vi "OdometricNavigation.vi"(0 "Wheel Angles (rad)":T3 {"RR Angle (rad)" scale=3.1416..-3.1416; "RL Angle (rad)" scale=3.1416..-3.1416; "FR Angle (rad)" scale=3.1416..-3.1416; "FL Angle (rad)" scale=3.1416..-3.1416}, 1 "Wheel Movements (in.)":cluster{"FL":dbl, "FR":dbl, "RL":dbl, "RR":dbl} {"RR" scale=-70.0..70.0; "RL" scale=-70.0..70.0; "FR" scale=-70.0..70.0; "FL" scale=-70.0..70.0}, 2 "Robot angle (degrees)":dbl(knob) scale=180.0..-180.0, 3 "x and y error minimum (in.)":dbl, 4 "error minimum for rotation (rad)":dbl) -> (17 "movement":cluster{"sy":dbl, "sx":dbl, "rot.":dbl})   [LabVIEW 2014]
uses:
  <vilib>/Analysis/baseanly.llb/Mean (DBL).vi
  Robot Global Data.vi
  <vilib>/Analysis/NI_AALBase.lvlib
panel:
  out "unhandled error data":dbl[][](array[numeric])
  out "Wheel X movements":T1
  out "Wheel Y movements":T2
  out "1-side error rotation (rad)":dbl
  out "compared":cluster{"sy":dbl, "sx":dbl, "rot.":dbl}[](array[cluster])
  out "Right Error":bool
  out "Front Error":bool
  out "Rear Error":bool
  out "Left Error":bool
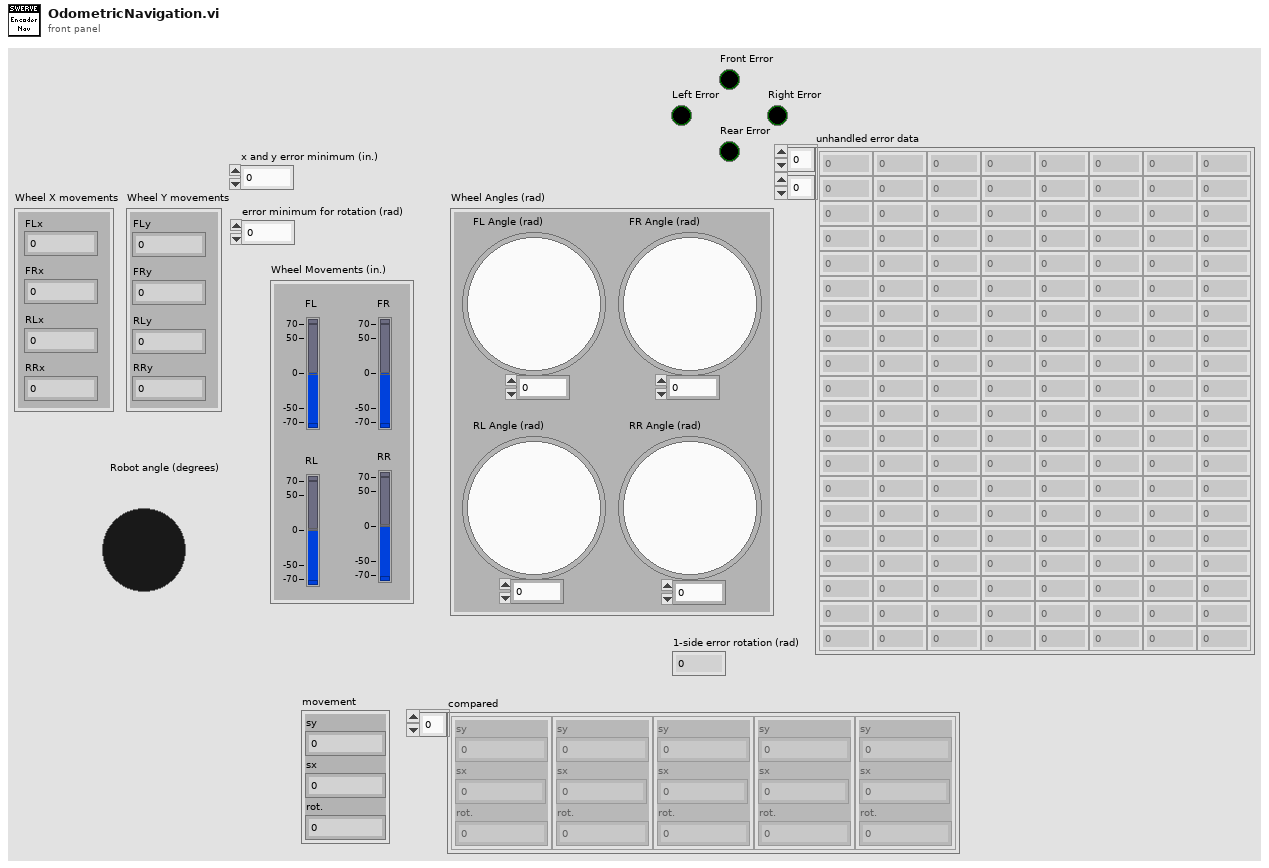
[diagram p1: front panel]
types:
  T1 = cluster{"FLx":dbl, "FRx":dbl, "RLx":dbl, "RRx":dbl}
  T2 = cluster{"FLy":dbl, "FRy":dbl, "RLy":dbl, "RRy":dbl}
  T3 = cluster{"FL Angle (rad)":dbl, "FR Angle (rad)":dbl, "RL Angle (rad)":dbl, "RR Angle (rad)":dbl}
  T4 = cluster{"[0]":dbl, "[1]":dbl, "[2]":dbl, "[3]":dbl}
  T5 = enum16{"no error", "front", "rear", "left", "right", "FL", "FR", "RL", "RR", "other"}
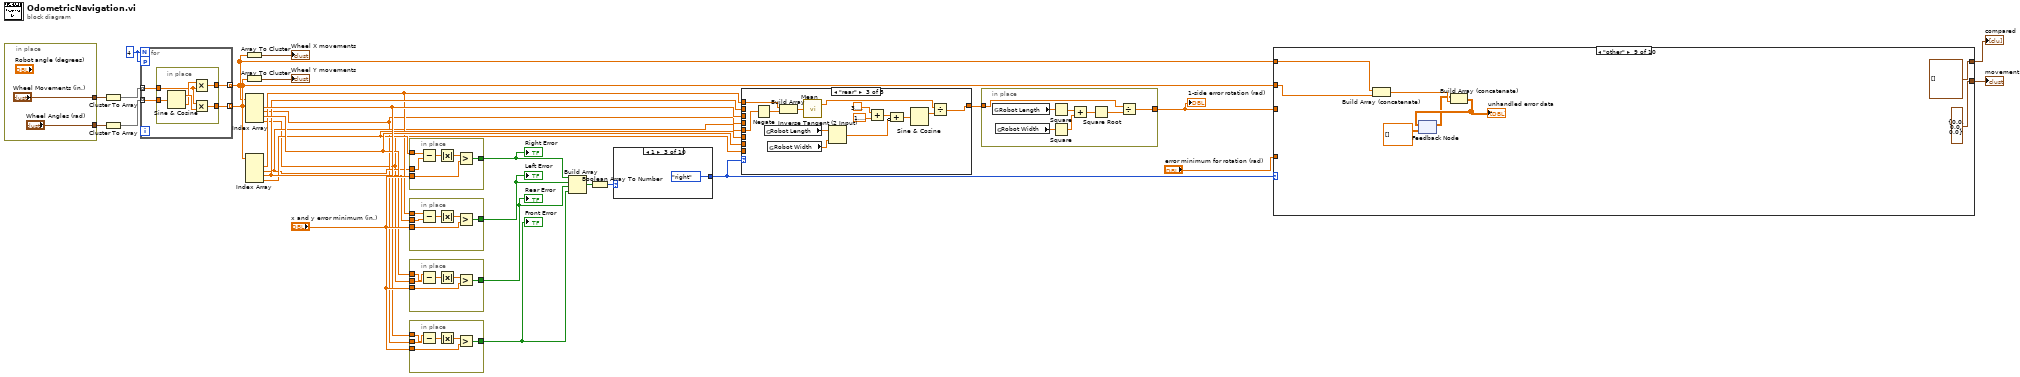
[diagram p0: block diagram]
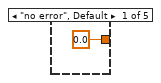
[diagram p2: hidden frame]
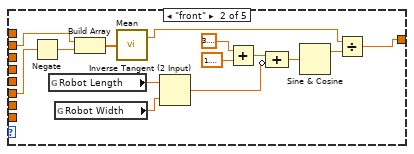
[diagram p3: hidden frame]
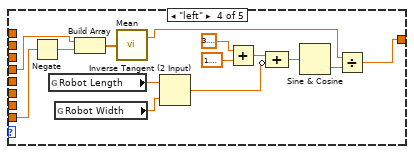
[diagram p4: hidden frame]
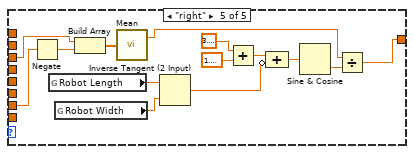
[diagram p5: hidden frame]
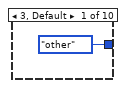
[diagram p6: hidden frame]
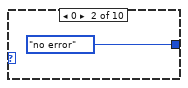
[diagram p7: hidden frame]
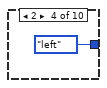
[diagram p8: hidden frame]
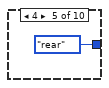
[diagram p9: hidden frame]
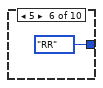
[diagram p10: hidden frame]
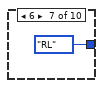
[diagram p11: hidden frame]
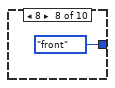
[diagram p12: hidden frame]
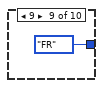
[diagram p13: hidden frame]
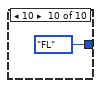
[diagram p14: hidden frame]
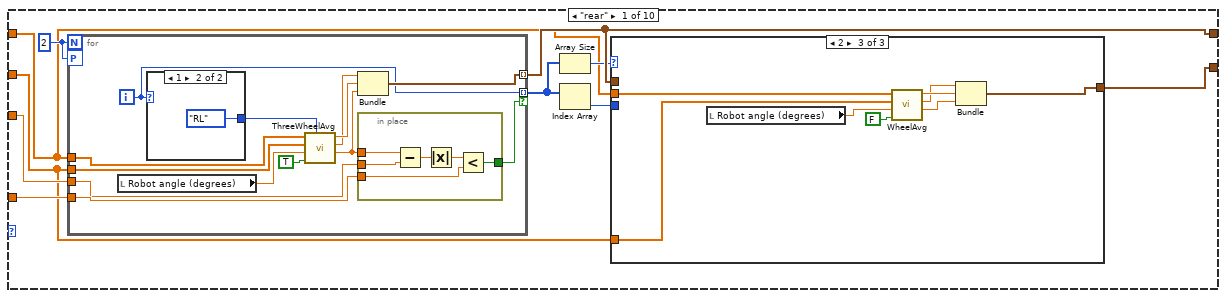
[diagram p15: hidden frame]
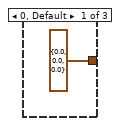
[diagram p16: hidden frame]
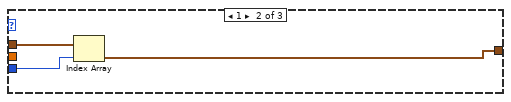
[diagram p17: hidden frame]
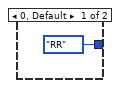
[diagram p18: hidden frame]
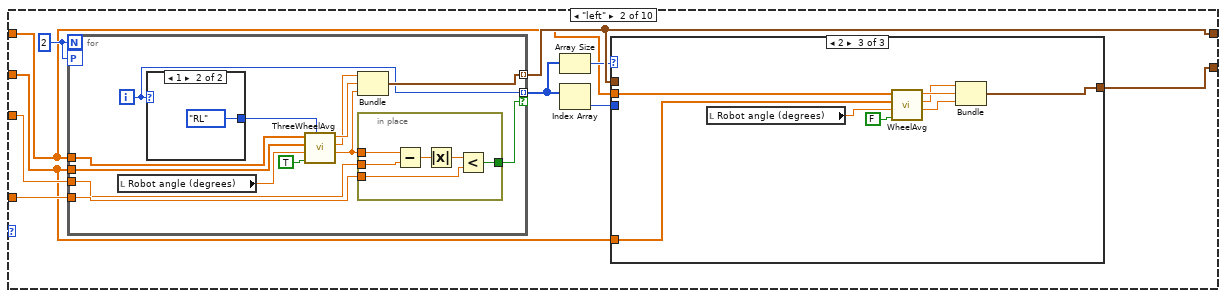
[diagram p19: hidden frame]
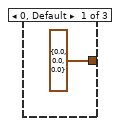
[diagram p20: hidden frame]
diagram:
  w16 = 4
  n1 = in-place {
    in-place-border: ["Wheel Movements (in.)"] -> w19
    in-place-border: ["Wheel Angles (rad)"] -> w18
  }
  n2 = Cluster To Array(cluster=w19) -> (array=w20:dbl[])
  n3 = Cluster To Array(cluster=w18) -> (array=w17:dbl[])
  n4 = for {
    N: w16 -> [_]
    tunnel: w20 -> [w36] mode=indexing
    tunnel: w17 -> [w35] mode=indexing
    workers-P: w16 -> [_]
    tunnel: [w34] -> w3 mode=indexing
    tunnel: [w33] -> w2 mode=indexing
    n5 = in-place {
      in-place-border: [w40] -> w33
      in-place-border: [w39] -> w34
      in-place-border: w36 -> [w38]
      in-place-border: w35 -> [w37]
      n6 = Sine & Cosine(0:w37) -> (1:w42:dbl, 2:w41:dbl)
      n7 = Multiply(x=w41, y=w38) -> (x*y=w40:dbl)
      n8 = Multiply(x=w38, y=w42) -> (x*y=w39:dbl)
    }
  }
  n9 = Array To Cluster(array=w2) -> (cluster=→"Wheel X movements":T4)
  n10 = Array To Cluster(array=w3) -> (cluster=→"Wheel Y movements":T4)
  n11 = Index Array(array=w2) -> (element #1=w12:dbl, element #2=w6:dbl, element #3=w11:dbl, element #4=w5:dbl)  [unwired: 4 in]
  n12 = Index Array(array=w3) -> (element #1=w8:dbl, element #2=w7:dbl, element #3=w10:dbl, element #4=w9:dbl)  [unwired: 4 in]
  n13 = in-place {
    in-place-border: [w46] -> w24
    in-place-border: w9 -> [w45]
    in-place-border: w7 -> [w44]
    in-place-border: "x and y error minimum (in.)" -> [w43]
    n14 = Subtract(x=w45, y=w44) -> (x-y=w48:dbl)
    n15 = Absolute Value(x=w48) -> (abs(x)=w47:dbl)
    n16 = Greater?(x=w47, y=w43) -> (0:w46:bool)
  }
  "Right Error" <- w24
  n17 = in-place {
    in-place-border: [w52] -> w21
    in-place-border: w8 -> [w51]
    in-place-border: w10 -> [w50]
    in-place-border: "x and y error minimum (in.)" -> [w49]
    n18 = Subtract(x=w51, y=w50) -> (x-y=w54:dbl)
    n19 = Absolute Value(x=w54) -> (abs(x)=w53:dbl)
    n20 = Greater?(x=w53, y=w49) -> (0:w52:bool)
  }
  "Left Error" <- w21
  n21 = in-place {
    in-place-border: [w58] -> w22
    in-place-border: w5 -> [w57]
    in-place-border: w11 -> [w56]
    in-place-border: "x and y error minimum (in.)" -> [w55]
    n22 = Subtract(x=w57, y=w56) -> (x-y=w60:dbl)
    n23 = Absolute Value(x=w60) -> (abs(x)=w59:dbl)
    n24 = Greater?(x=w59, y=w55) -> (0:w58:bool)
  }
  "Rear Error" <- w22
  n25 = in-place {
    in-place-border: [w64] -> w23
    in-place-border: w6 -> [w63]
    in-place-border: w12 -> [w62]
    in-place-border: "x and y error minimum (in.)" -> [w61]
    n26 = Subtract(x=w63, y=w62) -> (x-y=w66:dbl)
    n27 = Absolute Value(x=w66) -> (abs(x)=w65:dbl)
    n28 = Greater?(x=w65, y=w61) -> (0:w64:bool)
  }
  "Front Error" <- w23
  n29 = Build Array(w24, w21, w22, w23) -> (w26:bool[])
  n30 = Boolean Array To Number(Boolean array=w26) -> (number=w25:u32)
  n31 = case shown="1" w25 {
    tunnel: [T5."other" T5."no error" T5."right" T5."left" T5."rear" T5."RR" T5."RL" T5."front" T5."FR" T5."FL"] -> w13
    frame 3, Default {
    }
    frame 0 {
    }
    frame 1 {
    }
    frame 2 {
    }
    frame 4 {
    }
    frame 5 {
    }
    frame 6 {
    }
    frame 8 {
    }
    frame 9 {
    }
    frame 10 {
    }
  }
  n32 = case shown="\"rear\"" w13 {
    tunnel: [0.0 w80 w92 w106 w122] -> w4
    tunnel: w12 -> [_ _ _ _ w121]
    tunnel: w11 -> [_ _ _ _ w120]
    tunnel: w10 -> [_ w79 _ _ _]
    tunnel: w9 -> [_ w78 _ _ _]
    tunnel: w8 -> [_ _ w95 _ _]
    tunnel: w7 -> [_ _ w94 _ _]
    tunnel: w6 -> [_ _ _ w108 _]
    tunnel: w5 -> [_ _ _ w107 _]
    frame "no error", Default {
    }
    frame "front" {
      n33 = Negate(x=w78) -> (-x=w90:dbl)
      n34 = global read "Robot Global Data.vi" "Robot Length"() -> (w83:dbl)
      n35 = global read "Robot Global Data.vi" "Robot Width"() -> (w84:dbl)
      n36 = Build Array(w79, w90) -> (w91:dbl[])
      n37 = call-poly <vilib>:"Mean.vi"("X"=w91) -> ("mean"=w89:dbl)  [unwired: 1 out]
      n38 = Inverse Tangent (2 Input)(1:w84, 2:w83) -> (0:w85:dbl)
      n39 = Add(x=3.141592653589793, y=1.5707963267948966) -> (x+y=w86:dbl)
      n40 = Compound Arithmetic op=ADD(w86, invert w85) -> (w82:dbl)
      n41 = Sine & Cosine(0:w82) -> (1:w81:dbl)  [unwired: 1 out]
      n42 = Divide(x=w89, y=w81) -> (x/y=w80:dbl)
    }
    frame "rear" {
      n43 = Negate(x=w94) -> (-x=w104:dbl)
      n44 = global read "Robot Global Data.vi" "Robot Length"() -> (w98:dbl)
      n45 = global read "Robot Global Data.vi" "Robot Width"() -> (w99:dbl)
      n46 = Build Array(w95, w104) -> (w105:dbl[])
      n47 = call-poly <vilib>:"Mean.vi"("X"=w105) -> ("mean"=w103:dbl)  [unwired: 1 out]
      n48 = Inverse Tangent (2 Input)(1:w99, 2:w98) -> (0:w93:dbl)
      n49 = Add(x=3.141592653589793, y=1.5707963267948966) -> (x+y=w100:dbl)
      n50 = Compound Arithmetic op=ADD(w100, invert w93) -> (w97:dbl)
      n51 = Sine & Cosine(0:w97) -> (1:w96:dbl)  [unwired: 1 out]
      n52 = Divide(x=w103, y=w96) -> (x/y=w92:dbl)
    }
    frame "left" {
      n53 = Negate(x=w107) -> (-x=w118:dbl)
      n54 = global read "Robot Global Data.vi" "Robot Length"() -> (w111:dbl)
      n55 = global read "Robot Global Data.vi" "Robot Width"() -> (w112:dbl)
      n56 = Build Array(w108, w118) -> (w119:dbl[])
      n57 = call-poly <vilib>:"Mean.vi"("X"=w119) -> ("mean"=w117:dbl)  [unwired: 1 out]
      n58 = Inverse Tangent (2 Input)(1:w112, 2:w111) -> (0:w113:dbl)
      n59 = Add(x=3.141592653589793, y=1.5707963267948966) -> (x+y=w114:dbl)
      n60 = Compound Arithmetic op=ADD(w114, invert w113) -> (w110:dbl)
      n61 = Sine & Cosine(0:w110) -> (2:w109:dbl)  [unwired: 1 out]
      n62 = Divide(x=w117, y=w109) -> (x/y=w106:dbl)
    }
    frame "right" {
      n63 = Negate(x=w120) -> (-x=w132:dbl)
      n64 = global read "Robot Global Data.vi" "Robot Length"() -> (w126:dbl)
      n65 = global read "Robot Global Data.vi" "Robot Width"() -> (w127:dbl)
      n66 = Build Array(w121, w132) -> (w133:dbl[])
      n67 = call-poly <vilib>:"Mean.vi"("X"=w133) -> ("mean"=w124:dbl)  [unwired: 1 out]
      n68 = Inverse Tangent (2 Input)(1:w127, 2:w126) -> (0:w128:dbl)
      n69 = Add(x=3.141592653589793, y=1.5707963267948966) -> (x+y=w129:dbl)
      n70 = Compound Arithmetic op=ADD(w129, invert w128) -> (w125:dbl)
      n71 = Sine & Cosine(0:w125) -> (2:w123:dbl)  [unwired: 1 out]
      n72 = Divide(x=w124, y=w123) -> (x/y=w122:dbl)
    }
  }
  n73 = in-place {
    in-place-border: w4 -> [w135]
    in-place-border: [w134] -> w1
    n74 = global read "Robot Global Data.vi" "Robot Length"() -> (w141:dbl)
    n75 = global read "Robot Global Data.vi" "Robot Width"() -> (w140:dbl)
    n76 = Square(x=w141) -> (x^2=w138:dbl)
    n77 = Square(x=w140) -> (x^2=w139:dbl)
    n78 = Add(x=w138, y=w139) -> (x+y=w137:dbl)
    n79 = Square Root(x=w137) -> (sqrt(x)=w136:dbl)
    n80 = Divide(x=w135, y=w136) -> (x/y=w134:dbl)
  }
  "1-side error rotation (rad)" <- w1
  n81 = case shown="\"other\"" w13 {
    tunnel: [w147 w190 w233 w276 cluster{"mean":dbl, "mean":dbl, "mean":dbl}[] [] cluster{"mean":dbl, "mean":dbl, "mean":dbl}[] [] cluster{"mean":dbl, "mean":dbl, "mean":dbl}[] [] cluster{"mean":dbl, "mean":dbl, "mean":dbl}[] [] cluster{"mean":dbl, "mean":dbl, "mean":dbl}[] [] cluster{"mean":dbl, "mean":dbl, "mean":dbl}[] []] -> w29
    tunnel: "error minimum for rotation (rad)" -> [w151 w194 w237 w280 _ _ _ _ _ _]
    tunnel: [w148 w191 w234 w277 w323 w333 w343 w353 cluster{"mean":dbl, "mean":dbl, "mean":dbl} {"mean"=0.0, "mean"=0.0, "mean"=0.0} w369] -> w27
    tunnel: w3 -> [w143 w186 w229 w272 w319 w329 w339 w349 w358 w364]
    tunnel: w2 -> [w142 w185 w228 w271 w318 w328 w338 w348 w359 w363]
    tunnel: w1 -> [w146 w189 w232 w275 _ _ _ _ _ _]
    frame "rear" {
      w145 = 2
      n82 = for {
        N: w145 -> [_]
        tunnel: [w176] -> w147 mode=indexing
        tunnel: w151 -> [w175]
        tunnel: [w174] -> w150 mode=indexing if=w173
        tunnel: w143 -> [w170]
        tunnel: w142 -> [w169]
        tunnel: w146 -> [w164]
        workers-P: w145 -> [_]
        i -> [w174]
        n83 = local read "Robot angle (degrees)"() -> (w171:dbl)
        n84 = case shown="1" w174 {
          tunnel: [enum16{"FL", "FR", "RL", "RR"}."RR" ("Wheel Missing") enum16{"FL", "FR", "RL", "RR"}."RL" ("Wheel Missing")] -> w168
          frame 0, Default {
          }
          frame 1 {
          }
        }
        n85 = call "ThreeWheelAvg.vi"("Wheel Missing"=w168, "Calculate Rotation?"=TRUE, "Robot Angle (degrees)"=w171, "wheel Y movements (FL, FR, RL, RR)"=w170, "wheel X movements (FL, FR, RL, RR)"=w169) -> ("Rotation"=w165:dbl, "Y"=w166:dbl, "X"=w167:dbl)  [unwired: 4 in]
        n86 = Bundle("Y"=w166, "X"=w167, "Rotation"=w165) -> (w176:cluster{"Y":dbl, "X":dbl, "Rotation":dbl})  [unwired: 1 in]
        n87 = in-place {
          in-place-border: [w180] -> w173
          in-place-border: w175 -> [w179]
          in-place-border: w165 -> [w178]
          in-place-border: w164 -> [w177]
          n88 = Subtract(x=w178, y=w177) -> (x-y=w182:dbl)
          n89 = Absolute Value(x=w182) -> (abs(x)=w181:dbl)
          n90 = Less?(x=w181, y=w179) -> (x < y?=w180:bool)
        }
      }
      n91 = Array Size(array=w150) -> (size(s)=w144:i32)
      n92 = Index Array(array=w150) -> (element=w149:i32)  [unwired: 1 in]
      n93 = case shown="2" w144 {
        tunnel: w149 -> [_ w153 _]
        tunnel: [cluster{"Y":dbl, "X":dbl, "Rotation":dbl} {"Y"=0.0, "X"=0.0, "Rotation"=0.0} w155 w158] -> w148
        tunnel: w147 -> [_ w154 _]
        tunnel: w143 -> [_ _ w163]
        tunnel: w142 -> [_ _ w162]
        frame 0, Default {
        }
        frame 1 {
          n94 = Index Array(array=w154, index=w153) -> (element=w155:cluster{"Y":dbl, "X":dbl, "Rotation":dbl})
        }
        frame 2 {
          n95 = local read "Robot angle (degrees)"() -> (w156:dbl)
          n96 = call "WheelAvg.vi"("Calculate Rotation?"=FALSE, "Robot Angle (degrees)"=w156, "wheel Y movements (FL, FR, RL, RR)"=w163, "wheel X movements (FL, FR, RL, RR)"=w162) -> ("Rotation"=w159:dbl, "Y"=w160:dbl, "X"=w161:dbl)  [unwired: 5 in]
          n97 = Bundle("Y"=w160, "X"=w161, "Rotation"=w159) -> (w158:cluster{"Y":dbl, "X":dbl, "Rotation":dbl})  [unwired: 1 in]
        }
      }
    }
    frame "left" {
      w188 = 2
      n98 = for {
        N: w188 -> [_]
        tunnel: [w219] -> w190 mode=indexing
        tunnel: w194 -> [w218]
        tunnel: [w217] -> w193 mode=indexing if=w216
        tunnel: w186 -> [w213]
        tunnel: w185 -> [w212]
        tunnel: w189 -> [w207]
        workers-P: w188 -> [_]
        i -> [w217]
        n99 = local read "Robot angle (degrees)"() -> (w214:dbl)
        n100 = case shown="1" w217 {
          tunnel: [enum16{"FL", "FR", "RL", "RR"}."RR" ("Wheel Missing") enum16{"FL", "FR", "RL", "RR"}."RL" ("Wheel Missing")] -> w211
          frame 0, Default {
          }
          frame 1 {
          }
        }
        n101 = call "ThreeWheelAvg.vi"("Wheel Missing"=w211, "Calculate Rotation?"=TRUE, "Robot Angle (degrees)"=w214, "wheel Y movements (FL, FR, RL, RR)"=w213, "wheel X movements (FL, FR, RL, RR)"=w212) -> ("Rotation"=w208:dbl, "Y"=w209:dbl, "X"=w210:dbl)  [unwired: 4 in]
        n102 = Bundle("Y"=w209, "X"=w210, "Rotation"=w208) -> (w219:cluster{"Y":dbl, "X":dbl, "Rotation":dbl})  [unwired: 1 in]
        n103 = in-place {
          in-place-border: [w223] -> w216
          in-place-border: w218 -> [w222]
          in-place-border: w208 -> [w221]
          in-place-border: w207 -> [w220]
          n104 = Subtract(x=w221, y=w220) -> (x-y=w225:dbl)
          n105 = Absolute Value(x=w225) -> (abs(x)=w224:dbl)
          n106 = Less?(x=w224, y=w222) -> (x < y?=w223:bool)
        }
      }
      n107 = Array Size(array=w193) -> (size(s)=w187:i32)
      n108 = Index Array(array=w193) -> (element=w192:i32)  [unwired: 1 in]
      n109 = case shown="2" w187 {
        tunnel: w192 -> [_ w196 _]
        tunnel: [cluster{"Y":dbl, "X":dbl, "Rotation":dbl} {"Y"=0.0, "X"=0.0, "Rotation"=0.0} w198 w201] -> w191
        tunnel: w190 -> [_ w197 _]
        tunnel: w186 -> [_ _ w206]
        tunnel: w185 -> [_ _ w205]
        frame 0, Default {
        }
        frame 1 {
          n110 = Index Array(array=w197, index=w196) -> (element=w198:cluster{"Y":dbl, "X":dbl, "Rotation":dbl})
        }
        frame 2 {
          n111 = local read "Robot angle (degrees)"() -> (w199:dbl)
          n112 = call "WheelAvg.vi"("Calculate Rotation?"=FALSE, "Robot Angle (degrees)"=w199, "wheel Y movements (FL, FR, RL, RR)"=w206, "wheel X movements (FL, FR, RL, RR)"=w205) -> ("Rotation"=w202:dbl, "Y"=w203:dbl, "X"=w204:dbl)  [unwired: 5 in]
          n113 = Bundle("Y"=w203, "X"=w204, "Rotation"=w202) -> (w201:cluster{"Y":dbl, "X":dbl, "Rotation":dbl})  [unwired: 1 in]
        }
      }
    }
    frame "right" {
      w231 = 2
      n114 = for {
        N: w231 -> [_]
        tunnel: [w262] -> w233 mode=indexing
        tunnel: w237 -> [w261]
        tunnel: [w260] -> w236 mode=indexing if=w259
        tunnel: w229 -> [w256]
        tunnel: w228 -> [w255]
        tunnel: w232 -> [w250]
        workers-P: w231 -> [_]
        i -> [w260]
        n115 = local read "Robot angle (degrees)"() -> (w257:dbl)
        n116 = case shown="1" w260 {
          tunnel: [enum16{"FL", "FR", "RL", "RR"}."RR" ("Wheel Missing") enum16{"FL", "FR", "RL", "RR"}."RL" ("Wheel Missing")] -> w254
          frame 0, Default {
          }
          frame 1 {
          }
        }
        n117 = call "ThreeWheelAvg.vi"("Wheel Missing"=w254, "Calculate Rotation?"=TRUE, "Robot Angle (degrees)"=w257, "wheel Y movements (FL, FR, RL, RR)"=w256, "wheel X movements (FL, FR, RL, RR)"=w255) -> ("Rotation"=w251:dbl, "Y"=w252:dbl, "X"=w253:dbl)  [unwired: 4 in]
        n118 = Bundle("Y"=w252, "X"=w253, "Rotation"=w251) -> (w262:cluster{"Y":dbl, "X":dbl, "Rotation":dbl})  [unwired: 1 in]
        n119 = in-place {
          in-place-border: [w266] -> w259
          in-place-border: w261 -> [w265]
          in-place-border: w251 -> [w264]
          in-place-border: w250 -> [w263]
          n120 = Subtract(x=w264, y=w263) -> (x-y=w268:dbl)
          n121 = Absolute Value(x=w268) -> (abs(x)=w267:dbl)
          n122 = Less?(x=w267, y=w265) -> (x < y?=w266:bool)
        }
      }
      n123 = Array Size(array=w236) -> (size(s)=w230:i32)
      n124 = Index Array(array=w236) -> (element=w235:i32)  [unwired: 1 in]
      n125 = case shown="2" w230 {
        tunnel: w235 -> [_ w239 _]
        tunnel: [cluster{"Y":dbl, "X":dbl, "Rotation":dbl} {"Y"=0.0, "X"=0.0, "Rotation"=0.0} w241 w244] -> w234
        tunnel: w233 -> [_ w240 _]
        tunnel: w229 -> [_ _ w249]
        tunnel: w228 -> [_ _ w248]
        frame 0, Default {
        }
        frame 1 {
          n126 = Index Array(array=w240, index=w239) -> (element=w241:cluster{"Y":dbl, "X":dbl, "Rotation":dbl})
        }
        frame 2 {
          n127 = local read "Robot angle (degrees)"() -> (w242:dbl)
          n128 = call "WheelAvg.vi"("Calculate Rotation?"=FALSE, "Robot Angle (degrees)"=w242, "wheel Y movements (FL, FR, RL, RR)"=w249, "wheel X movements (FL, FR, RL, RR)"=w248) -> ("Rotation"=w245:dbl, "Y"=w246:dbl, "X"=w247:dbl)  [unwired: 5 in]
          n129 = Bundle("Y"=w246, "X"=w247, "Rotation"=w245) -> (w244:cluster{"Y":dbl, "X":dbl, "Rotation":dbl})  [unwired: 1 in]
        }
      }
    }
    frame "front" {
      w274 = 2
      n130 = for {
        N: w274 -> [_]
        tunnel: [w305] -> w276 mode=indexing
        tunnel: w280 -> [w304]
        tunnel: [w303] -> w279 mode=indexing if=w302
        tunnel: w272 -> [w299]
        tunnel: w271 -> [w298]
        tunnel: w275 -> [w293]
        workers-P: w274 -> [_]
        i -> [w303]
        n131 = local read "Robot angle (degrees)"() -> (w300:dbl)
        n132 = case shown="1" w303 {
          tunnel: [enum16{"FL", "FR", "RL", "RR"}."RR" ("Wheel Missing") enum16{"FL", "FR", "RL", "RR"}."RL" ("Wheel Missing")] -> w297
          frame 0, Default {
          }
          frame 1 {
          }
        }
        n133 = call "ThreeWheelAvg.vi"("Wheel Missing"=w297, "Calculate Rotation?"=TRUE, "Robot Angle (degrees)"=w300, "wheel Y movements (FL, FR, RL, RR)"=w299, "wheel X movements (FL, FR, RL, RR)"=w298) -> ("Rotation"=w294:dbl, "Y"=w295:dbl, "X"=w296:dbl)  [unwired: 4 in]
        n134 = Bundle("Y"=w295, "X"=w296, "Rotation"=w294) -> (w305:cluster{"Y":dbl, "X":dbl, "Rotation":dbl})  [unwired: 1 in]
        n135 = in-place {
          in-place-border: [w309] -> w302
          in-place-border: w304 -> [w308]
          in-place-border: w294 -> [w307]
          in-place-border: w293 -> [w306]
          n136 = Subtract(x=w307, y=w306) -> (x-y=w311:dbl)
          n137 = Absolute Value(x=w311) -> (abs(x)=w310:dbl)
          n138 = Less?(x=w310, y=w308) -> (x < y?=w309:bool)
        }
      }
      n139 = Array Size(array=w279) -> (size(s)=w273:i32)
      n140 = Index Array(array=w279) -> (element=w278:i32)  [unwired: 1 in]
      n141 = case shown="2" w273 {
        tunnel: w278 -> [_ w282 _]
        tunnel: [cluster{"Y":dbl, "X":dbl, "Rotation":dbl} {"Y"=0.0, "X"=0.0, "Rotation"=0.0} w284 w287] -> w277
        tunnel: w276 -> [_ w283 _]
        tunnel: w272 -> [_ _ w292]
        tunnel: w271 -> [_ _ w291]
        frame 0, Default {
        }
        frame 1 {
          n142 = Index Array(array=w283, index=w282) -> (element=w284:cluster{"Y":dbl, "X":dbl, "Rotation":dbl})
        }
        frame 2 {
          n143 = local read "Robot angle (degrees)"() -> (w285:dbl)
          n144 = call "WheelAvg.vi"("Calculate Rotation?"=FALSE, "Robot Angle (degrees)"=w285, "wheel Y movements (FL, FR, RL, RR)"=w292, "wheel X movements (FL, FR, RL, RR)"=w291) -> ("Rotation"=w288:dbl, "Y"=w289:dbl, "X"=w290:dbl)  [unwired: 5 in]
          n145 = Bundle("Y"=w289, "X"=w290, "Rotation"=w288) -> (w287:cluster{"Y":dbl, "X":dbl, "Rotation":dbl})  [unwired: 1 in]
        }
      }
    }
    frame "FL" {
      # "fl"
      n146 = local read "Robot angle (degrees)"() -> (w321:dbl)
      n147 = call "ThreeWheelAvg.vi"("Wheel Missing"=enum16{"FL", "FR", "RL", "RR"}."FL", "Calculate Rotation?"=FALSE, "Robot Angle (degrees)"=w321, "wheel Y movements (FL, FR, RL, RR)"=w319, "wheel X movements (FL, FR, RL, RR)"=w318) -> ("Rotation"=w315:dbl, "Y"=w314:dbl, "X"=w316:dbl)  [unwired: 4 in]
      n148 = Bundle("Y"=w314, "X"=w316, "Rotation"=w315) -> (w323:cluster{"Y":dbl, "X":dbl, "Rotation":dbl})  [unwired: 1 in]
    }
    frame "FR" {
      # "fl"
      n149 = local read "Robot angle (degrees)"() -> (w331:dbl)
      n150 = call "ThreeWheelAvg.vi"("Wheel Missing"=enum16{"FL", "FR", "RL", "RR"}."FR", "Calculate Rotation?"=FALSE, "Robot Angle (degrees)"=w331, "wheel Y movements (FL, FR, RL, RR)"=w329, "wheel X movements (FL, FR, RL, RR)"=w328) -> ("Rotation"=w325:dbl, "Y"=w324:dbl, "X"=w326:dbl)  [unwired: 4 in]
      n151 = Bundle("Y"=w324, "X"=w326, "Rotation"=w325) -> (w333:cluster{"Y":dbl, "X":dbl, "Rotation":dbl})  [unwired: 1 in]
    }
    frame "RL" {
      # "fl"
      n152 = local read "Robot angle (degrees)"() -> (w341:dbl)
      n153 = call "ThreeWheelAvg.vi"("Wheel Missing"=enum16{"FL", "FR", "RL", "RR"}."RL", "Calculate Rotation?"=FALSE, "Robot Angle (degrees)"=w341, "wheel Y movements (FL, FR, RL, RR)"=w339, "wheel X movements (FL, FR, RL, RR)"=w338) -> ("Rotation"=w335:dbl, "Y"=w334:dbl, "X"=w336:dbl)  [unwired: 4 in]
      n154 = Bundle("Y"=w334, "X"=w336, "Rotation"=w335) -> (w343:cluster{"Y":dbl, "X":dbl, "Rotation":dbl})  [unwired: 1 in]
    }
    frame "RR" {
      # "fl"
      n155 = local read "Robot angle (degrees)"() -> (w351:dbl)
      n156 = call "ThreeWheelAvg.vi"("Wheel Missing"=enum16{"FL", "FR", "RL", "RR"}."RR", "Calculate Rotation?"=FALSE, "Robot Angle (degrees)"=w351, "wheel Y movements (FL, FR, RL, RR)"=w349, "wheel X movements (FL, FR, RL, RR)"=w348) -> ("Rotation"=w345:dbl, "Y"=w344:dbl, "X"=w346:dbl)  [unwired: 4 in]
      n157 = Bundle("Y"=w344, "X"=w346, "Rotation"=w345) -> (w353:cluster{"Y":dbl, "X":dbl, "Rotation":dbl})  [unwired: 1 in]
    }
    frame "other" {
      n158 = Build Array (concatenate)(w359, w358) -> (w357:dbl[])
      n159 = feedback #1(dbl[][] []) -> (w355:dbl[][])
      n160 = Build Array (concatenate)(w355, w357) -> (w356:dbl[][])
      "unhandled error data" <- w356
      n161 = feedback-in #1(w356) -> ()
    }
    frame "no error" {
      n162 = local read "Robot angle (degrees)"() -> (w362:dbl)
      n163 = call "WheelAvg.vi"("Calculate Rotation?"=FALSE, "Robot Angle (degrees)"=w362, "wheel Y movements (FL, FR, RL, RR)"=w364, "wheel X movements (FL, FR, RL, RR)"=w363) -> ("Rotation"=w366:dbl, "Y"=w367:dbl, "X"=w368:dbl)  [unwired: 5 in]
      n164 = Bundle("Y"=w367, "X"=w368, "Rotation"=w366) -> (w369:cluster{"Y":dbl, "X":dbl, "Rotation":dbl})  [unwired: 1 in]
    }
  }
  "compared" <- w29
  "movement" <- w27
